vi "Setting.vi"() -> ()   [LabVIEW 2020]
uses:
  Global_Variable/Global.vi
panel:
  in  "右工位扭矩偏移":cluster{"正向":dbl, "逆向":dbl} {"逆向" format="%#.2f Nm"; "正向" format="%#.2f Nm"}
  in  "左工位扭矩偏移":cluster{"正向":dbl, "逆向":dbl} {"逆向" format="%#.2f Nm"; "正向" format="%#.2f Nm"}
  # "配置标定"
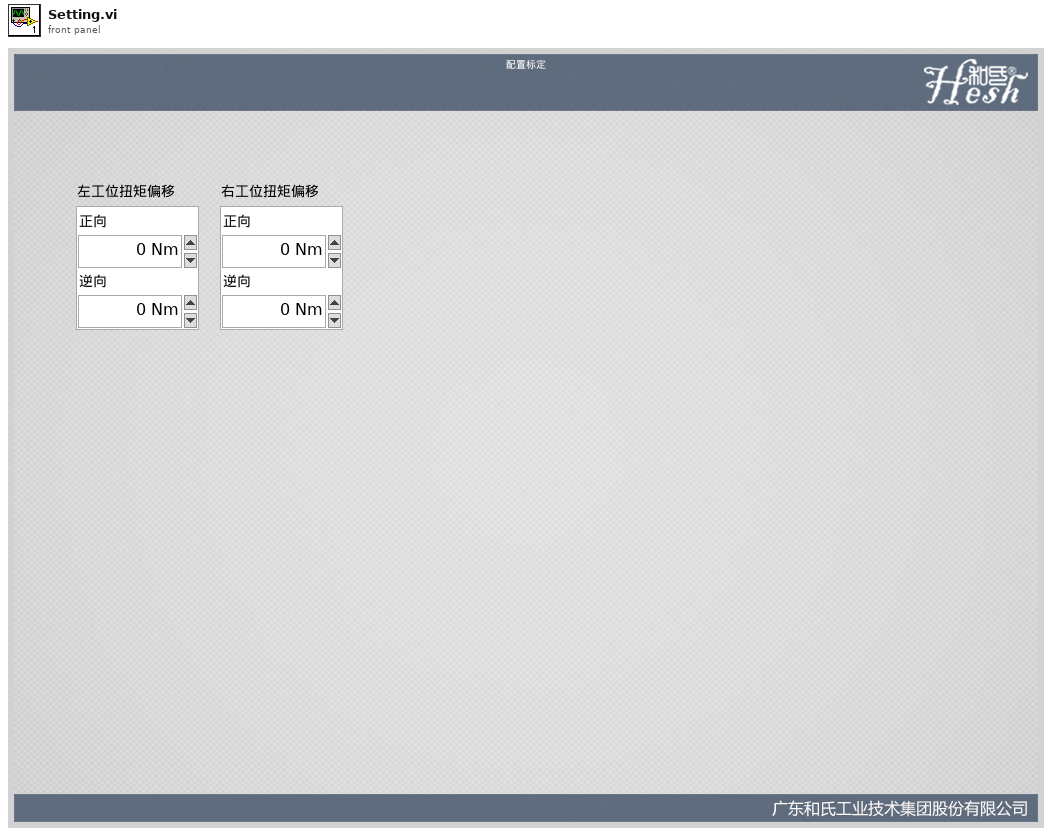
[diagram p1: front panel]
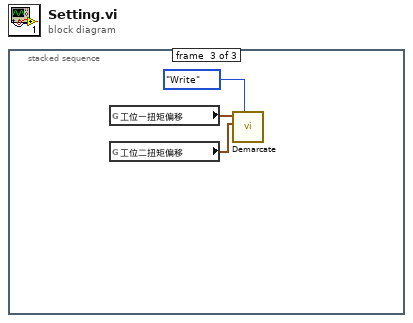
[diagram p0: block diagram]
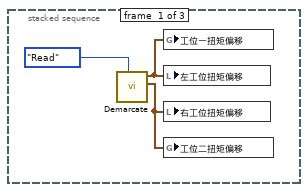
[diagram p2: hidden frame]
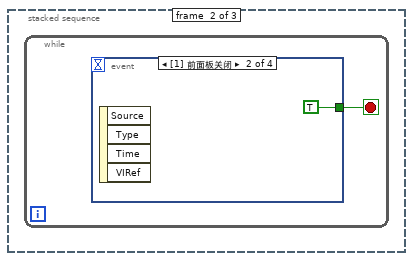
[diagram p3: hidden frame]
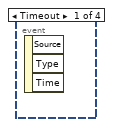
[diagram p4: hidden frame]
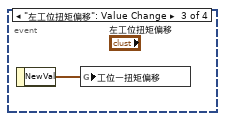
[diagram p5: hidden frame]
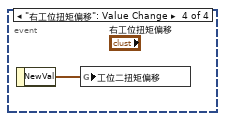
[diagram p6: hidden frame]
diagram:
  n1 = stacked-sequence {
    frame #0 {
      n2 = call "Demarcate.vi"("Mode"=enum16{"Read", "Write"}."Read") -> ("工位二扭矩偏移O"=w1:cluster{"正向":dbl, "逆向":dbl}, "工位一扭矩偏移O"=w2:cluster{"正向":dbl, "逆向":dbl})  [unwired: 8 in, 1 out]
      n3 = global write "Global.vi" "工位一扭矩偏移"(w2) -> ()
      n4 = local write "左工位扭矩偏移"(w2) -> ()
      n5 = local write "右工位扭矩偏移"(w1) -> ()
      n6 = global write "Global.vi" "工位二扭矩偏移"(w1) -> ()
    }
    frame #1 {
      n7 = while {
        stop <- w4 stop-if-true
        n8 = event shown="[1] 前面板关闭" {
          selector: _ -> [_ _ _ _]
          dyn-events: _ -> [_ _ _ _]
          timeout: _ -> [_ _ _ _]
          tunnel: [_ TRUE _ _] -> w4
          event Timeout {
            n9 = event-data() -> ()  [unwired: 1 in, 3 out]
          }
          event Panel Close {
            n10 = event-data() -> ()  [unwired: 1 in, 4 out]
          }
          event "左工位扭矩偏移": Value Change {
            n11 = event-data() -> ("NewVal"=w6:cluster{"正向":dbl, "逆向":dbl})  [unwired: 1 in]
            n12 = global write "Global.vi" "工位一扭矩偏移"(w6) -> ()
          }
          event "右工位扭矩偏移": Value Change {
            n13 = event-data() -> ("NewVal"=w7:cluster{"正向":dbl, "逆向":dbl})  [unwired: 1 in]
            n14 = global write "Global.vi" "工位二扭矩偏移"(w7) -> ()
          }
        }
      }
    }
    frame #2 {
      n15 = global read "Global.vi" "工位一扭矩偏移"() -> (w9:cluster{"正向":dbl, "逆向":dbl})
      n16 = global read "Global.vi" "工位二扭矩偏移"() -> (w10:cluster{"正向":dbl, "逆向":dbl})
      n17 = call "Demarcate.vi"("Mode"=enum16{"Read", "Write"}."Write", "工位二扭矩偏移"=w10, "工位一扭矩偏移"=w9) -> ()  [unwired: 6 in, 3 out]
    }
  }
